vi "Create Block Terminals.vi"(8 "error in (no error)":errorcluster, 9 "Output?":bool, 10 "Inputs":string[](array[string]), 11 "Rectangle in":refnum<class "Rectangle.lvclass">) -> (0 "error out":errorcluster, 3 "Array":refnum<class "Terminal.lvclass">[](array[class]))   [LabVIEW 2015]
uses:
  Terminal Form/Terminal.lvclass
  <vilib>/LIEF/Forms/Rectangle/Rectangle.lvclass
  <vilib>/LIEF/Forms/Text/Text.lvclass
  <vilib>/LIEF/Forms/Shape/Shape.lvclass
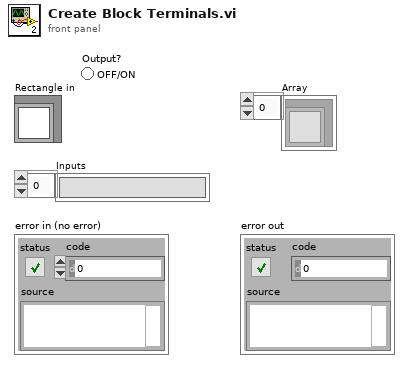
[diagram p1: front panel]
types:
  T1 = enum16{"Left", "Top", "Right", "Bottom", "Centered"}
  T2 = cluster{"Font Name:":string, "Size":i16, "Strikeout?":bool, "Italic?":bool, "Underline?":bool, "Outline?":bool, "Shadow?":bool, "Bold?":bool}
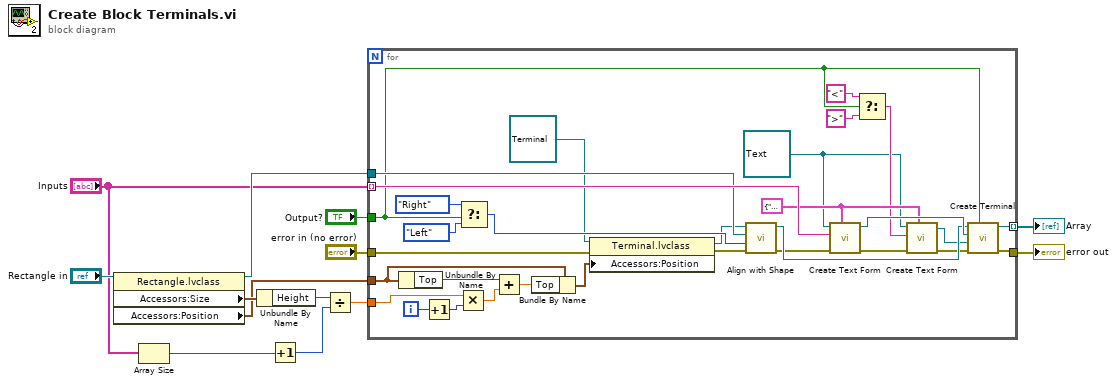
[diagram p0: block diagram]
diagram:
  n1 = property class="Rectangle.lvclass"(reference="Rectangle in") -> (reference out=w8:refnum<class "Rectangle.lvclass">, "Accessors:Size"=w7:cluster{"Width":i32, "Height":i32}, "Accessors:Position"=w2:cluster{"Left":i32, "Top":i32})  [unwired: 1 in, 1 out]
  n2 = Array Size(array="Inputs") -> (size(s)=w4:i32)
  n3 = Unbundle By Name(w7) -> ("Height"=w6:i32)
  n4 = Increment(x=w4) -> (x+1=w1:i32)
  n5 = Divide(x=w6, y=w1) -> (x/y=w3:dbl)
  n6 = for {
    tunnel: "Inputs" -> [w44] mode=indexing
    tunnel: "Output?" -> [w24]
    tunnel: w8 -> [w43]
    tunnel: [w32] -> w11 mode=indexing
    tunnel: "error in (no error)" -> [w15]
    tunnel: [w31] -> w13
    tunnel: w3 -> [w39]
    tunnel: w2 -> [w37]
    i -> [w34]
    w14 = refnum<class "Text.lvclass"> refnum ("Text in")
    w25 = T2 {"Font Name:"="Segoe UI", "Size"=15, "Strikeout?"=FALSE, "Italic?"=FALSE, "Underline?"=FALSE, "Outline?"=FALSE, "Shadow?"=FALSE, "Bold?"=FALSE} ("[user-specified font]")
    n7 = Unbundle By Name(w37) -> ("Top"=w35:i32)
    n8 = Increment(x=w34) -> (x+1=w33:i32)
    n9 = Multiply(x=w39, y=w33) -> (x*y=w38:dbl)
    n10 = Select(t=T1."Right" ("Alignment"), s=w24, f=T1."Left" ("Alignment")) -> (s? t:f=w40:T1)
    n11 = Add(x=w35, y=w38) -> (x+y=w36:dbl)
    n12 = Bundle By Name(cluster=w37, "Top"=w36) -> (w29:cluster{"Left":i32, "Top":i32})
    n13 = property class="Terminal.lvclass"(reference=refnum<class "Terminal.lvclass"> refnum ("Terminal in"), error in=w15, "Accessors:Position"=w29) -> (reference out=w28:refnum<class "Terminal.lvclass">, error out=w17:errorcluster)
    n14 = call <vilib>:"Align with Shape.vi"("error in (no error)"=w17, "Alignment"=w40, "Reference Shape"=w43, "Shape in"=w28) -> ("error out"=w16:errorcluster, "Shape out"=w26:refnum<class "Terminal.lvclass">)  [unwired: 6 in]
    n15 = call <vilib>:"Create Text Form.vi"("[user-specified font]"=w25, "error in (no error)"=w16, "Text"=w44, "Text in"=w14) -> ("error out"=w19:errorcluster, "New Text"=w27:refnum<class "Text.lvclass">)  [unwired: 6 in]
    n16 = Select(t="<", s=w24, f=">") -> (s? t:f=w21:string)
    n17 = call <vilib>:"Create Text Form.vi"("[user-specified font]"=w25, "error in (no error)"=w19, "Text"=w21, "Text in"=w14) -> ("error out"=w18:errorcluster, "New Text"=w20:refnum<class "Text.lvclass">)  [unwired: 6 in]
    n18 = call "Create Terminal.vi"("Direction"=w24, "error in (no error)"=w18, "Symbol"=w20, "Text Shape"=w27, "Terminal in"=w26) -> ("error out"=w31:errorcluster, "Terminal out"=w32:refnum<class "Terminal.lvclass">)  [unwired: 5 in]
  }
  "error out" <- w13
  "Array" <- w11
